vi "Stop Core.vi"(10 "final error code":i32, 11 "Automation Controller in":refnum<class "Automation Controller.lvclass">) -> (3 "Automation Controller out":refnum<class "Automation Controller.lvclass">)   [LabVIEW 2024]
doc: "<p>(<strong>Filename</strong>: <span class=\"dnl\">Actor Framework.lvlib:Actor.lvclass:Stop Core.vi</span>)</p>\n<p>Defines what the actor does before it stops. Use the <strong>final error code</strong> input to determine whether the actor shut down in response to an error.</p>\n<p>By default, this method passes the Stop message along to all <a href=\"nihelplauncher://docs/csh?context=lvcore_lvcomm_af_launch_nested_actor\">auto-stop nested actors</a>. A descendant class may override this method to define additional behavior, such as shutting down any processes the actor initiated in its override of the <a href=\"nihelplauncher://docs/csh?context=lvcore_lvcomm_af_actor_core\">Actor Core</a> method.</p>"
uses:
  Automation Controller.lvclass/Automation Controller.ctl
  Automation Controller.lvclass
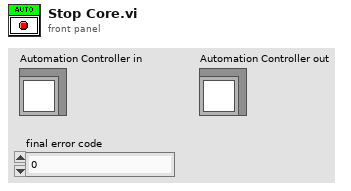
[diagram p1: front panel]
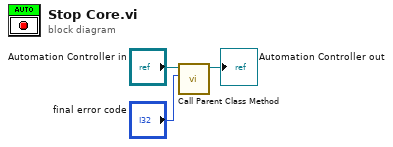
[diagram p0: block diagram]
diagram:
  n1 = call-parent "Call Parent Class Method"("final error code"="final error code", "Actor in"="Automation Controller in") -> ("Actor out"=→"Automation Controller out":refnum<class "Automation Controller.lvclass">)  [unwired: 9 in]
